vi "ImageClickDetect v1.0 .vi"(7 "Stop":refnum<vi>, 9 "Mouse Point":refnum<vi>, 11 "image Ref String":string) -> ()   [LabVIEW 2016]
panel:
  out "ImXY_Point":i32[](array[numeric])
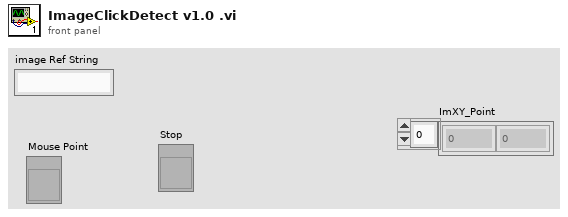
[diagram p1: front panel]
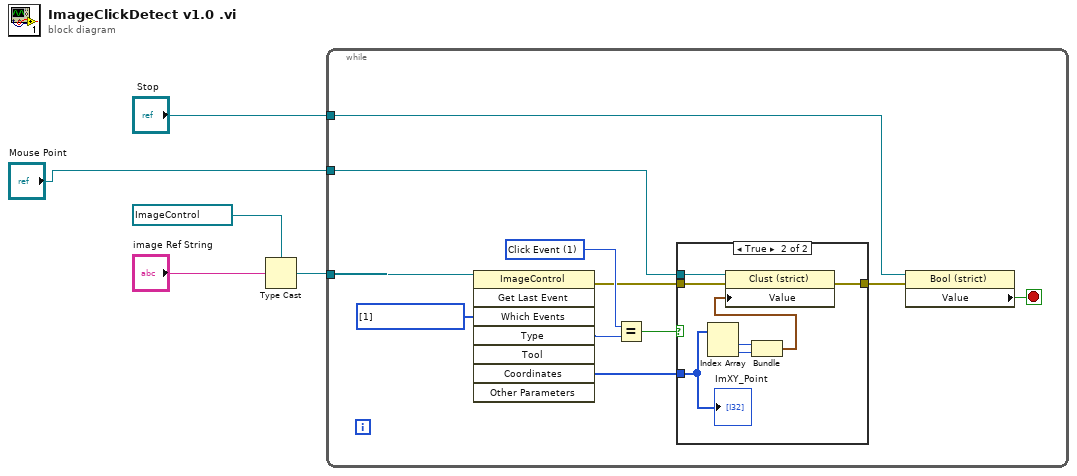
[diagram p0: block diagram]
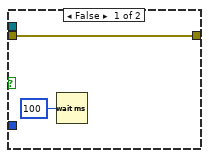
[diagram p2: hidden frame]
diagram:
  n1 = Type Cast(type=refnum<vi> refnum ("Image"), x="image Ref String") -> (*(type *) &x=w3:refnum<vi>)
  n2 = while {
    tunnel: w3 -> [w16]
    tunnel: "Stop" -> [w10]
    tunnel: "Mouse Point" -> [w8]
    stop <- w9 stop-if-true
    w13 = 1 items=["No Event"=0, "Click Event"=1, "Draw Event"=2, "Size Event"=4, "Scroll Event"=5, "Double Click Event"=8]
    w15 = i32[] [1] items=["No Event"=0, "Click Event"=1, "Draw Event"=2, "Size Event"=4, "Scroll Event"=5, "Double Click Event"=8] ("Which Events")
    n3 = invoke class="ImageControl" method="Get Last Event"(reference=w16, "Which Events"=w15) -> (error out=w7:errorcluster, "Type"=w14:i32, "Coordinates"=w11:i32[])  [unwired: 6 in, 5 out]
    n4 = Equal?(x=w13, y=w14) -> (x = y?=w12:bool)
    n5 = case shown="True" w12 {
      tunnel: w11 -> [_ w21]
      tunnel: w8 -> [_ w25]
      tunnel: w7 -> [w17 w24]
      tunnel: [w17 w23] -> w6
      frame False {
        n6 = Wait (ms)(milliseconds to wait=u32 100) -> ()  [unwired: 1 out]
      }
      frame True {
        n7 = Index Array(array=w21) -> (element #1=w20:i32, element #2=w19:i32)  [unwired: 2 in]
        n8 = Bundle(w20, w19) -> (w22:cluster{i32, i32})  [unwired: 1 in]
        n9 = property class="Clust (strict)"(reference=w25, error in=w24, "Value"=w22) -> (error out=w23:errorcluster)  [unwired: 1 out]
        "ImXY_Point" <- w21
      }
    }
    n10 = property class="Bool (strict)"(reference=w10, error in=w6) -> ("Value"=w9:bool)  [unwired: 2 out]
  }
